vi "Configure Streaming.vi"(8 "error in (no error)":errorcluster, 9 "Enable Streaming (Enable)":bool, 11 "VISA resource name":refnum<visa-resource-name>) -> (0 "error out":errorcluster, 3 "VISA resource name out":refnum<visa-resource-name>)   [LabVIEW 2015, in "Micron Optics sm130.lvlib"]
doc: "Configures the streaming mode for the instrument. During streaming mode, the instrument will generate the GET_DATA command internally. In order to extract data, only a read is required. The instrument will not respond to messages so that there is no desynchronization of the data that is being passed.\n\nIf a Read VI besides the Read Streaming Data is run, there will be an error. Therefore, disable streaming mode before using the other read vi's."
uses:
  Micron Optics sm130.lvlib
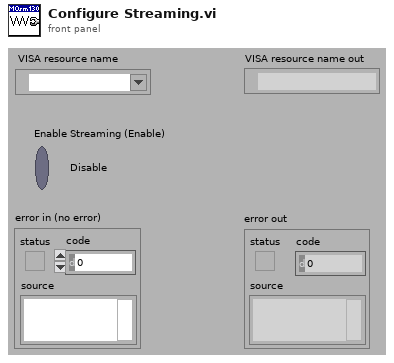
[diagram p1: front panel]
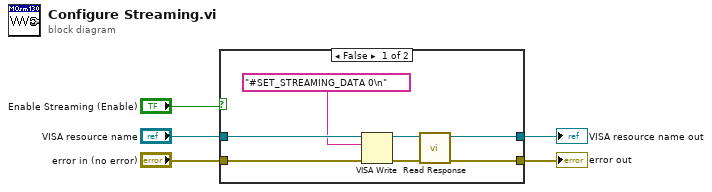
[diagram p0: block diagram]
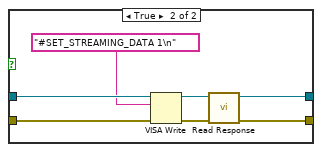
[diagram p2: hidden frame]
diagram:
  n1 = case shown="False" "Enable Streaming (Enable)" {
    tunnel: "VISA resource name" -> [w12 w19]
    tunnel: [w7 w14] -> w3
    tunnel: [w6 w13] -> w2
    tunnel: "error in (no error)" -> [w11 w18]
    frame False {
      n2 = VISA Write(VISA resource name=w12, write buffer="#SET_STREAMING_DATA 0\n", error in (no error)=w11) -> (VISA resource name out=w9:refnum<visa-resource-name>, error out=w8:errorcluster)  [unwired: 1 out]
      n3 = call "Read Response.vi"("error in (no error)"=w8, "VISA resource name"=w9) -> ("error out"=w6:errorcluster, "VISA resource name out"=w7:refnum<visa-resource-name>)  [unwired: 7 in, 1 out]
    }
    frame True {
      n4 = VISA Write(VISA resource name=w19, write buffer="#SET_STREAMING_DATA 1\n", error in (no error)=w18) -> (VISA resource name out=w16:refnum<visa-resource-name>, error out=w15:errorcluster)  [unwired: 1 out]
      n5 = call "Read Response.vi"("error in (no error)"=w15, "VISA resource name"=w16) -> ("error out"=w13:errorcluster, "VISA resource name out"=w14:refnum<visa-resource-name>)  [unwired: 7 in, 1 out]
    }
  }
  "VISA resource name out" <- w3
  "error out" <- w2
